vi "Main_17A.vi"() -> ()   [LabVIEW 2024]
uses:
  MAP_Registers.ctl
  ENUM_Instructions.ctl
  <vilib>/Utility/error.llb/Trim Whitespace One-Sided.vi
  Utility/Universal Utility/TypeDefs_Utility/Cluster_Row-Column.ctl
  ENUM_Combo Select.ctl
panel:
  out "Register start":T1
  out "Output":u64[](array[numeric])
  out "Register end":T1
  out "Answer":string
  in  "Select Data":T2(tab)
  in  "Example":string="Register A: 729\nRegister B: 0\nRegister C: 0\n\nProgram: 0,1,5,4,3,0"
  in  "Puzzle":string="Register A: 60589763\nRegister B: 0\nRegister C: 0\n\nProgram: 2,4,1,5,7,5,1,6,4,1,5,5,0,3,3,0"
  in  "Example A":string="Register A: 0\nRegister B: 0\nRegister C: 9\n\nProgram: 2,6"
  in  "Example B":string="Register A: 10\nRegister B: 0\nRegister C: 0\n\nProgram: 5,0,5,1,5,4"
  in  "Example C":string="Register A: 2024\nRegister B: 0\nRegister C: 0\n\nProgram: 0,1,5,4,3,0"
  in  "Example D":string="Register A: 0\nRegister B: 29\nRegister C: 0\n\nProgram: 1,7"
  in  "Example E":string="Register A: 0\nRegister B: 2024\nRegister C: 43690\n\nProgram: 4,0"
  out "Register Map":T1
  out "Program":i32[](array[numeric])
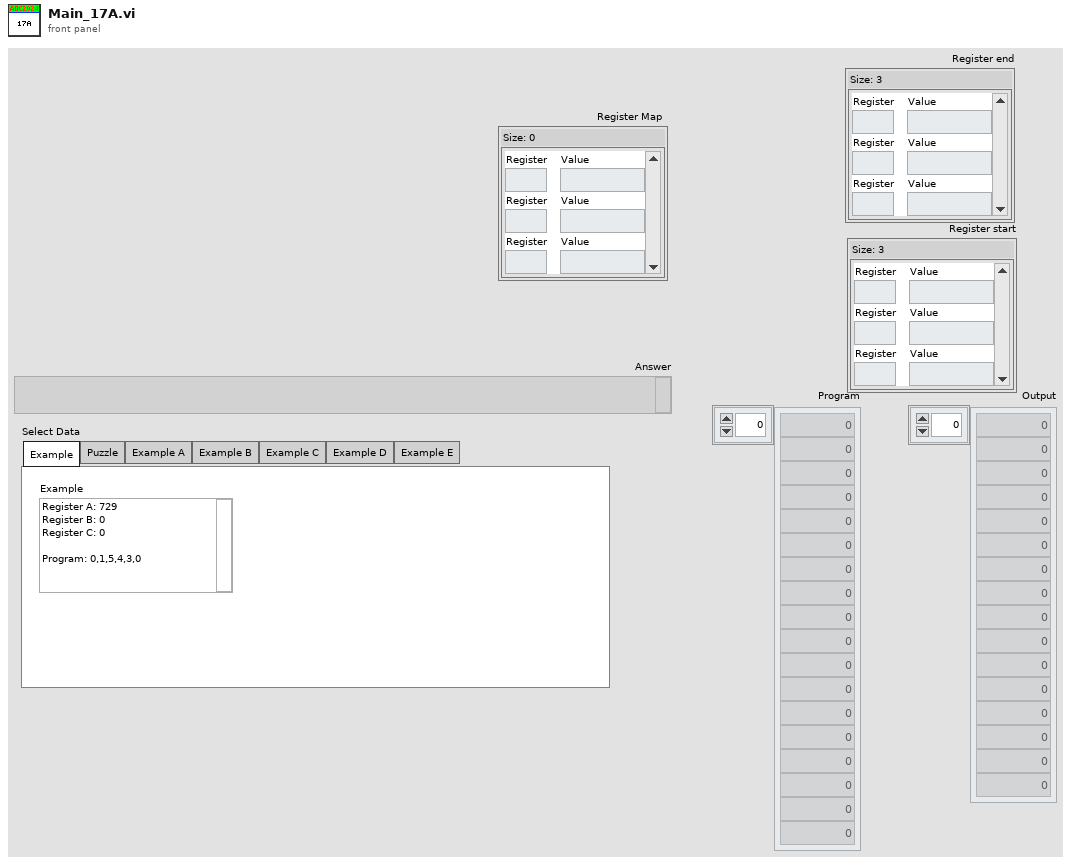
[diagram p1: front panel]
types:
  T1 = typedef "MAP_Registers.ctl" = map{string, i32}
  T2 = enum32{"Example", "Puzzle", "Example A", "Example B", "Example C", "Example D", "Example E"}
  T3 = typedef "ENUM_Instructions.ctl" = enum16{"adv: 0 [A/(2^combo)] Truncated TO A", "bxl: 1 [B XOR literal] TO B", "bst: 2 [combo MOD 8] TO B", "jnz: 3 [jump Pointer litteral]", "bxc: 4 [B XOR C] TO B", "out: 5 [combo MOD 8] TO OUT", "bdv: 6 [A/(2^combo)] Truncated TO B", "cdv: 7 [A/(2^combo)] Truncated TO C"}
  T4 = typedef "ENUM_Instructions.ctl" = enum16{"adv: [A/(2^combo)] Truncated TO A", "bxl: [B XOR literal] TO B", "bst: [combo MOD 8] TO B", "jnz: [jump Pointer litteral]", "bxc: [B XOR C] TO B", "out: [combo MOD 8] TO OUT", "bdv: [A/(2^combo)] Truncated TO B", "cdv:  [A/(2^combo)] Truncated TO C"}
  T5 = typedef "ENUM_Combo Select.ctl" = enum16{"0", "1", "2", "3", "A", "B", "C", "XXX"}
  T6 = typedef "Cluster_Row-Column.ctl" = cluster{"R":i32, "C":i32}
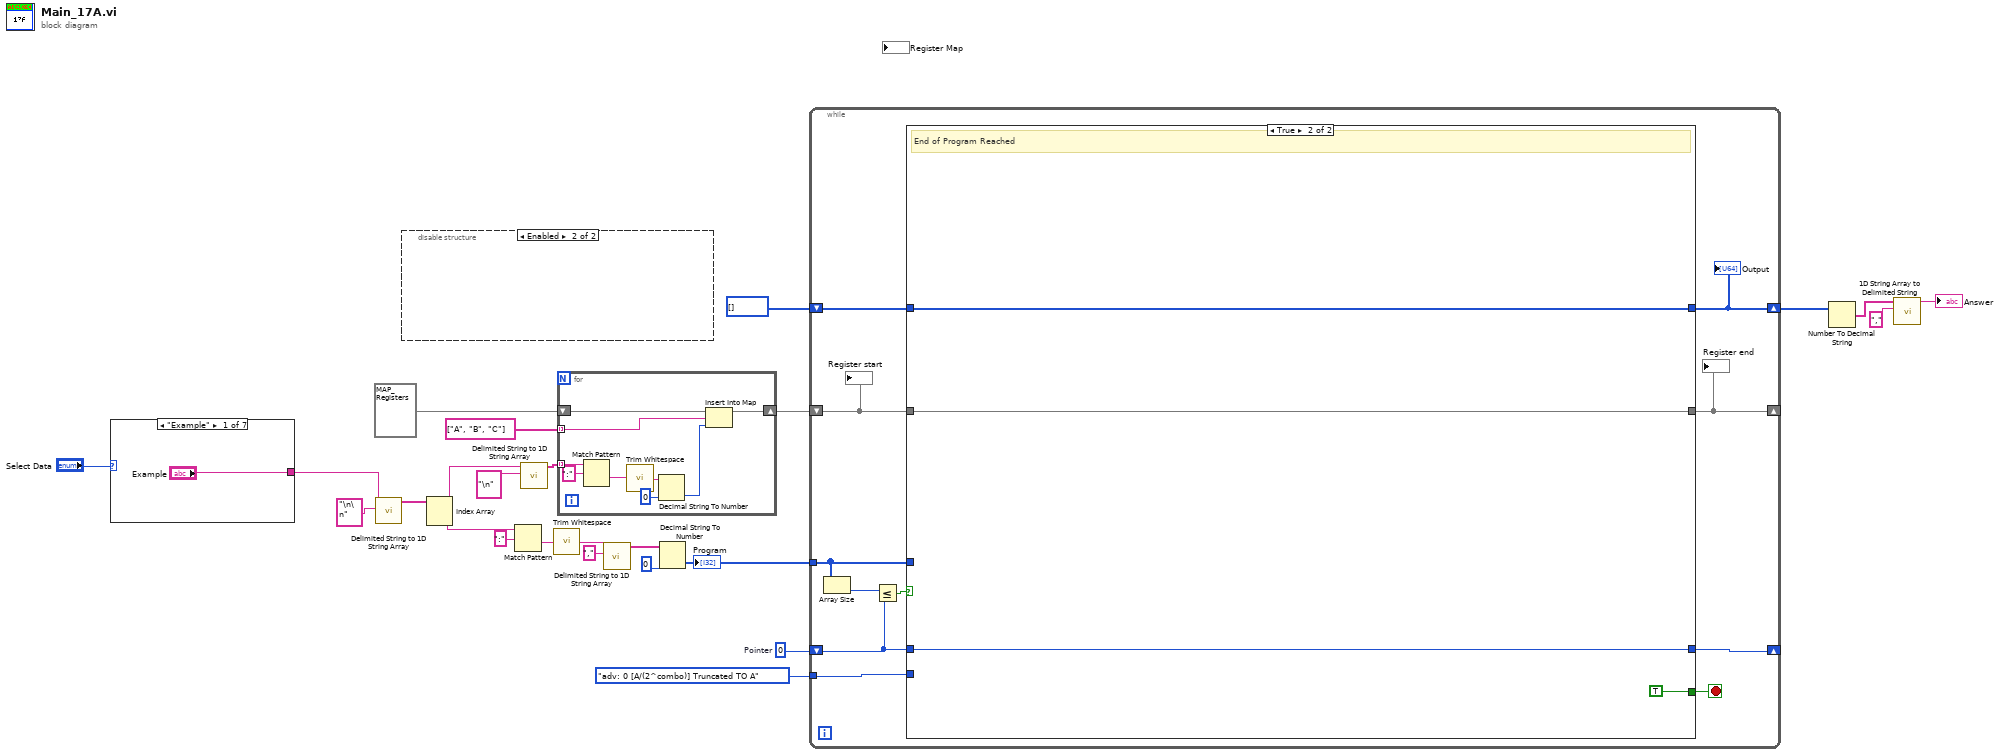
[diagram p0: block diagram]
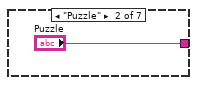
[diagram p2: hidden frame]
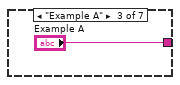
[diagram p3: hidden frame]
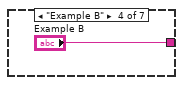
[diagram p4: hidden frame]
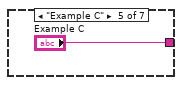
[diagram p5: hidden frame]
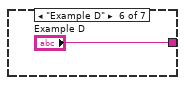
[diagram p6: hidden frame]
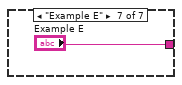
[diagram p7: hidden frame]
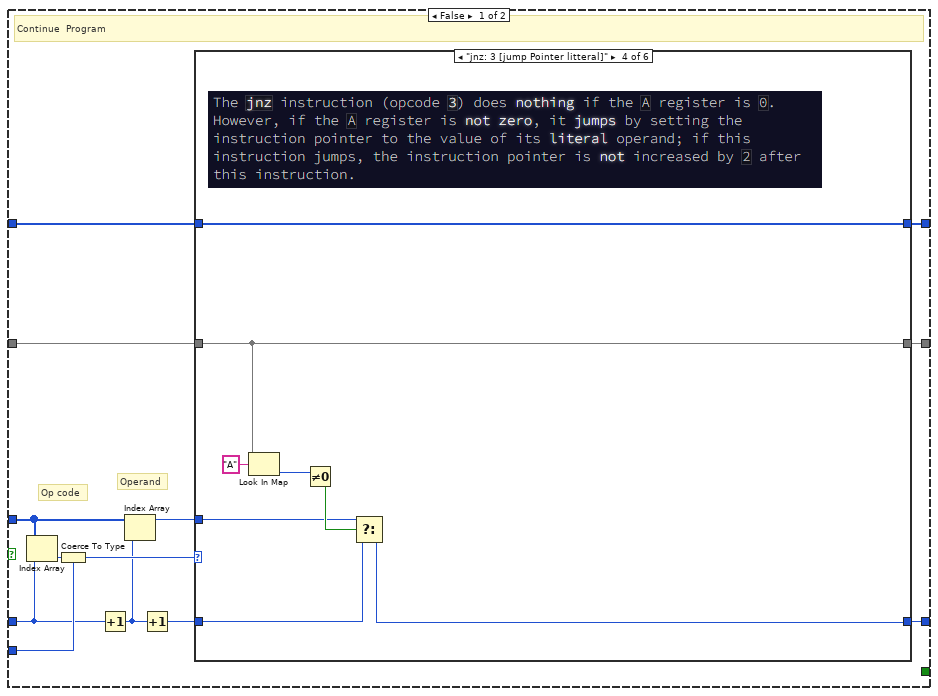
[diagram p8: hidden frame]
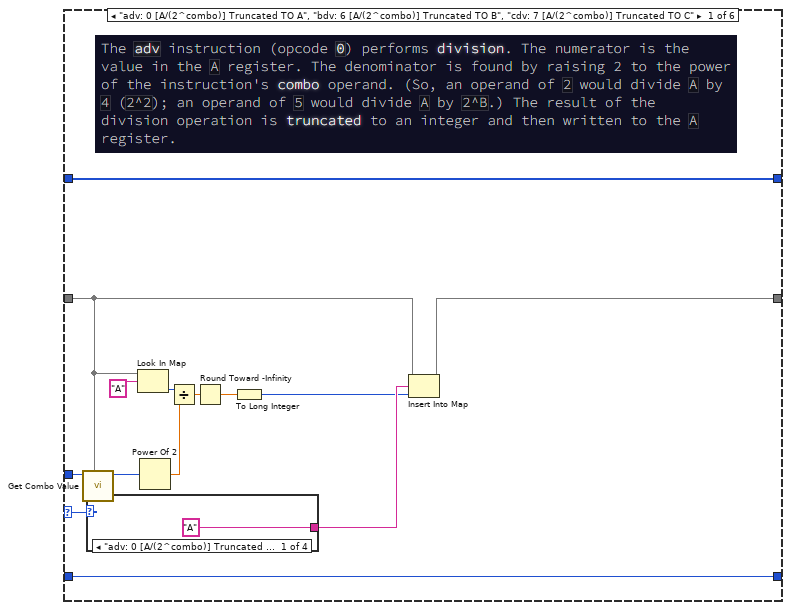
[diagram p9: hidden frame]
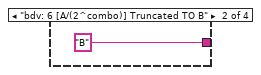
[diagram p10: hidden frame]
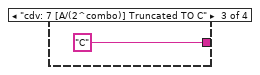
[diagram p11: hidden frame]
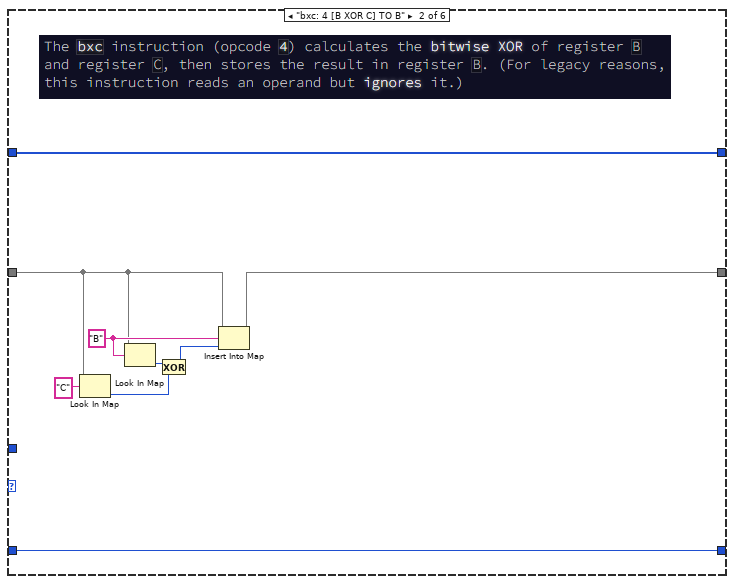
[diagram p13: hidden frame]
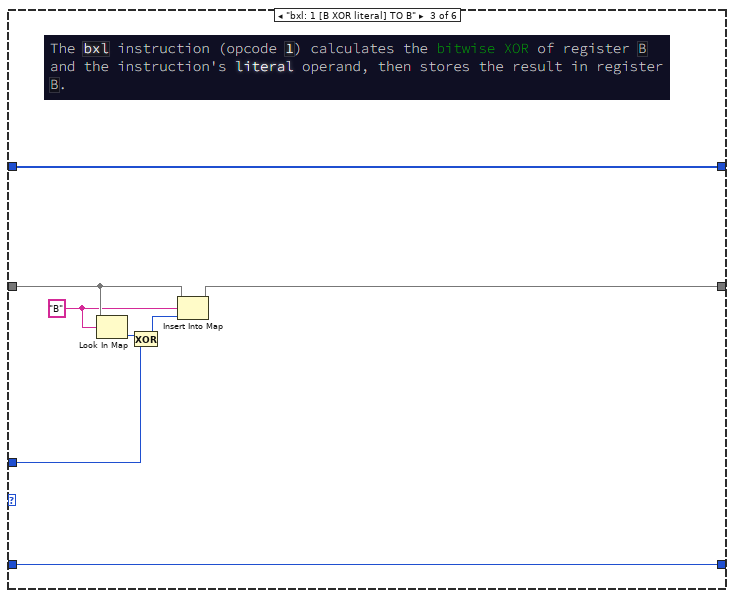
[diagram p14: hidden frame]
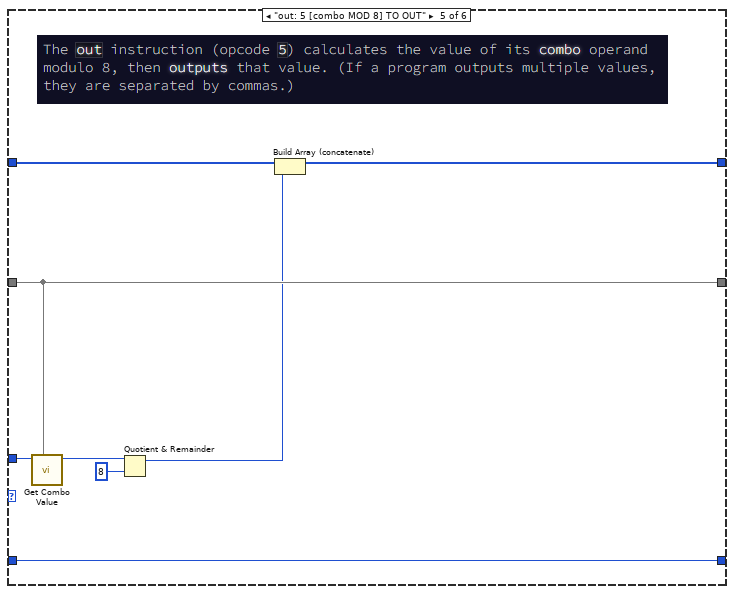
[diagram p15: hidden frame]
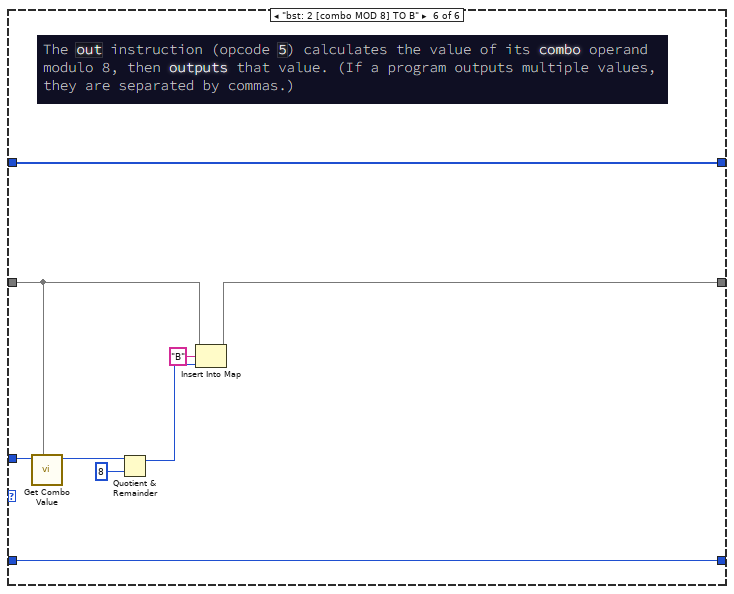
[diagram p16: hidden frame]
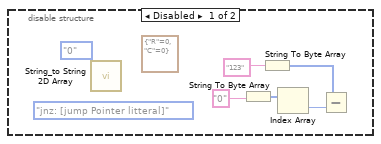
[diagram p17: hidden frame]
diagram:
  w9 = 0  # Pointer
  n1 = case shown="\"Example\"" "Select Data" {
    tunnel: ["Example" "Puzzle" "Example A" "Example B" "Example C" "Example D" "Example E"] -> w5
    frame "Example" {
    }
    frame "Puzzle" {
    }
    frame "Example A" {
    }
    frame "Example B" {
    }
    frame "Example C" {
    }
    frame "Example D" {
    }
    frame "Example E" {
    }
  }
  n2 = call <vilib>:"Delimited String to 1D String Array.vi"("delimiter"="\n\n" ("delimiter (Tab)"), "delimited string"=w5) -> ("string array"=w24:string[])  [unwired: 9 in]
  n3 = disable-structure shown="Enabled" {
    frame Disabled {
      (unwired) ENUM_Instructions."jnz: [jump Pointer litteral]" ("Instructions")
      (unwired) ENUM_Combo_Select."0" ("Combo")
      (unwired) T6 {"R"=0, "C"=0} ("Position")
      n4 = call "String_to String 2D Array.vi"() -> ()  [unwired: 11 in, 1 out]
      n5 = String To Byte Array(string="0") -> (unsigned byte array=w35:u8[])
      n6 = String To Byte Array(string="123") -> (unsigned byte array=w33:u8[])
      n7 = Index Array(array=w35) -> (element=w34:u8)  [unwired: 1 in]
      n8 = Subtract(x=w33, y=w34) -> ()  [unwired: 1 out]
    }
    frame Enabled {
    }
  }
  n9 = Index Array(array=w24) -> (element #1=w23:string, element #2=w18:string)  [unwired: 2 in]
  n10 = Match Pattern(string=w18, regular expression=":") -> (after substring=w16:string)  [unwired: 1 in, 3 out]
  n11 = call <vilib>:"Delimited String to 1D String Array.vi"("delimiter"="\n" ("delimiter (Tab)"), "delimited string"=w23) -> ("string array"=w21:string[])  [unwired: 9 in]
  n12 = call <vilib>:"Trim Whitespace.vi"("string"=w16) -> ("trimmed string"=w15:string)  [unwired: 1 in]
  n13 = for {
    tunnel: w21 -> [w46] mode=indexing
    shift-right: [w41] -> w11
    shift-left: T1 {} -> [w42]
    tunnel: string[] ["A", "B", "C"] ("String") -> [w40] mode=indexing
    n14 = Match Pattern(string=w46, regular expression=":") -> (after substring=w44:string)  [unwired: 1 in, 3 out]
    n15 = call <vilib>:"Trim Whitespace.vi"("string"=w44) -> ("trimmed string"=w43:string)  [unwired: 1 in]
    n16 = Decimal String To Number(string=w43, default (0L)=u64 0 ("default (0 I32)")) -> (number=w39:u64)  [unwired: 1 in, 1 out]
    n17 = Insert Into Map(map in=w42, key=w40, value=w39) -> (map out=w41:T1)  [unwired: 2 out]
  }
  n18 = call <vilib>:"Delimited String to 1D String Array.vi"("delimiter"=",", "delimited string"=w15) -> ("string array"=w13:string[])  [unwired: 9 in]
  n19 = Decimal String To Number(string=w13, default (0L)=0 ("default (0 I32)")) -> (number=w10:i32[])  [unwired: 1 in, 1 out]
  "Program" <- w10
  n20 = while {
    shift-right: [w49] -> _
    shift-left: w11 -> [w48]
    tunnel: w10 -> [w57]
    shift-right: [w52] -> _
    shift-left: w9 -> [w56]
    shift-right: [w47] -> w3
    shift-left: i32[] [] -> [w54]
    tunnel: ENUM_Instructions."adv: 0 [A/(2^combo)] Truncated TO A" ("Instructions") -> [w53]
    stop <- w51 stop-if-true
    n21 = Array Size(array=w57) -> (size(s)=w50:i32)
    n22 = Less Or Equal?(x=w50, y=w56) -> (x <= y?=w55:bool)
    n23 = case shown="True" w55 {
      tunnel: w57 -> [w60 _]
      tunnel: w56 -> [w63 w132]
      tunnel: w48 -> [w65 w131]
      tunnel: w54 -> [w67 w133]
      tunnel: w53 -> [w68 _]
      tunnel: [w66 w133] -> w47
      tunnel: [w58 w132] -> w52
      tunnel: [w64 w131] -> w49
      tunnel: [_ TRUE] -> w51
      frame False {
        # "Operand"
        # "Op code"
        # "Continue  Program"
        n24 = Index Array(array=w60, index=w63) -> (element=w70:i32)
        n25 = Coerce To Type(0:w70, 1:w68) -> (2:w69:T3)
        n26 = Increment(x=w63) -> (x+1=w62:i32)
        n27 = Index Array(array=w60, index=w62) -> (element=w61:i32)
        n28 = Increment(x=w62) -> (x+1=w59:i32)
        n29 = case shown="\"jnz: 3 [jump Pointer litteral]\"" w69 {
          selector: w69 -> [w75 _ _ _ _ _]
          tunnel: w61 -> [w82 _ w97 w107 w118 w127]
          tunnel: w67 -> [w84 w96 w104 w112 w120 w129]
          tunnel: [w84 w96 w104 w112 w114 w129] -> w66
          tunnel: w65 -> [w73 w90 w101 w111 w117 w123]
          tunnel: [w74 w94 w102 w111 w117 w124] -> w64
          tunnel: w59 -> [w83 w95 w103 w105 w119 w128]
          tunnel: [w83 w95 w103 w106 w119 w128] -> w58
          frame "adv: 0 [A/(2^combo)] Truncated TO A", "bdv: 6 [A/(2^combo)] Truncated TO B", "cdv: 7 [A/(2^combo)] Truncated TO C" {
            n30 = call "Get Combo Value.vi"("Register Map"=w73, "Operand"=w82) -> ("Combo Value"=w81:i32)  [unwired: 9 in]
            n31 = case shown="\"adv: 0 [A/(2^combo)] Truncated TO A\"" w75 {
              tunnel: ["A" ("key") "B" ("key") "C" ("key") _] -> w72
              frame "adv: 0 [A/(2^combo)] Truncated TO A" {
              }
              frame "bdv: 6 [A/(2^combo)] Truncated TO B" {
              }
              frame "cdv: 7 [A/(2^combo)] Truncated TO C" {
              }
              frame Default {
              }
            }
            n32 = Look In Map(map=w73, key="A") -> (value=w78:i32)  [unwired: 1 in, 1 out]
            n33 = Power Of 2(x=w81) -> (2^x=w79:dbl)
            n34 = Divide(x=w78, y=w79) -> (x/y=w77:dbl)
            n35 = Round Toward -Infinity(1:w77) -> (0:w76:dbl)
            n36 = To Long Integer(number=w76) -> (32bit integer=w71:i32)
            n37 = Insert Into Map(map in=w73, key=w72, value=w71) -> (map out=w74:T1)  [unwired: 2 out]
          }
          frame "bxc: 4 [B XOR C] TO B" {
            w93 = "B" ("key")
            n38 = Look In Map(map=w90, key="C") -> (value=w88:i32)  [unwired: 1 in, 1 out]
            n39 = Look In Map(map=w90, key=w93) -> (value=w92:i32)  [unwired: 1 in, 1 out]
            n40 = Exclusive Or(1:w88, 2:w92) -> (0:w91:i32)
            n41 = Insert Into Map(map in=w90, key=w93, value=w91) -> (map out=w94:T1)  [unwired: 2 out]
          }
          frame "bxl: 1 [B XOR literal] TO B" {
            w100 = "B" ("key")
            n42 = Look In Map(map=w101, key=w100) -> (value=w99:i32)  [unwired: 1 in, 1 out]
            n43 = Exclusive Or(1:w97, 2:w99) -> (0:w98:i32)
            n44 = Insert Into Map(map in=w101, key=w100, value=w98) -> (map out=w102:T1)  [unwired: 2 out]
          }
          frame "jnz: 3 [jump Pointer litteral]" {
            n45 = Look In Map(map=w111, key="A") -> (value=w109:i32)  [unwired: 1 in, 1 out]
            n46 = Not Equal To 0?(x=w109) -> (x != 0?=w108:bool)
            n47 = Select(t=w107, s=w108, f=w105) -> (s? t:f=w106:i32)
          }
          frame "out: 5 [combo MOD 8] TO OUT" {
            n48 = call "Get Combo Value.vi"("Register Map"=w117, "Operand"=w118) -> ("Combo Value"=w116:i32)  [unwired: 9 in]
            n49 = Quotient & Remainder(x=w116, y=8) -> (x-y*floor(x/y)=w113:i32)  [unwired: 1 out]
            n50 = Build Array (concatenate)(w120, w113) -> (w114:i32[])
          }
          frame "bst: 2 [combo MOD 8] TO B" {
            n51 = call "Get Combo Value.vi"("Register Map"=w123, "Operand"=w127) -> ("Combo Value"=w126:i32)  [unwired: 9 in]
            n52 = Quotient & Remainder(x=w126, y=8) -> (x-y*floor(x/y)=w121:i32)  [unwired: 1 out]
            n53 = Insert Into Map(map in=w123, key="B", value=w121) -> (map out=w124:T1)  [unwired: 2 out]
          }
        }
      }
      frame True {
        # "End of Program Reached"
      }
    }
    "Register end" <- w49
    "Output" <- w47
    "Register start" <- w48
  }
  n54 = Number To Decimal String(number=w3) -> (decimal integer string=w2:string[])  [unwired: 1 in]
  n55 = call <vilib>:"1D String Array to Delimited String.vi"("delimiter"=",", "string array"=w2) -> ("delimited string"=→"Answer":string)  [unwired: 9 in]
